vi "alu.vi"(2 "CONTROL":T3, 3 "INPUT_B":T2, 4 "INPUT_A":T2) -> (0 "OVERFLOW":bool, 1 "OUTPUT":T1)   [LabVIEW 2013]
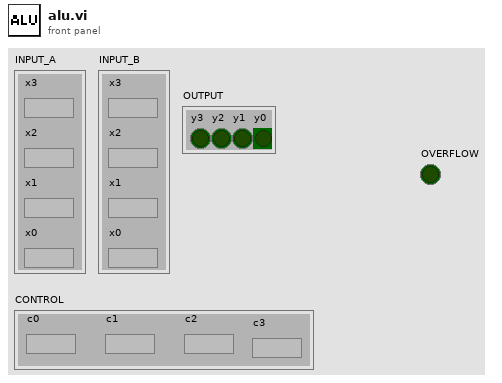
[diagram p1: front panel]
types:
  T1 = cluster{"y3":bool, "y2":bool, "y1":bool, "y0":bool}
  T2 = cluster{"x3":bool, "x2":bool, "x1":bool, "x0":bool}
  T3 = cluster{"с0":bool, "с1":bool, "с2":bool, "c3":bool}
  T4 = cluster{"y0":bool, "y1":bool, "y2":bool, "y3":bool}
  T5 = cluster{"INPUT_A":cluster{"x3":bool, "x2":bool, "x1":bool, "x0":bool}, cluster{"x3":bool, "x2":bool, "x1":bool, "x0":bool}, cluster{"x3":bool, "x2":bool, "x1":bool, "x0":bool}, cluster{"x3":bool, "x2":bool, "x1":bool, "x0":bool}, cluster{"x3":bool, "x2":bool, "x1":bool, "x0":bool}, "OUTPUT":cluster{"y3":bool, "y2":bool, "y1":bool, "y0":bool}, "OUTPUT":cluster{"y3":bool, "y2":bool, "y1":bool, "y0":bool}, "OUTPUT":cluster{"y0":bool, "y1":bool, "y2":bool, "y3":bool}, "OUTPUT":cluster{"y3":bool, "y2":bool, "y1":bool, "y0":bool}}
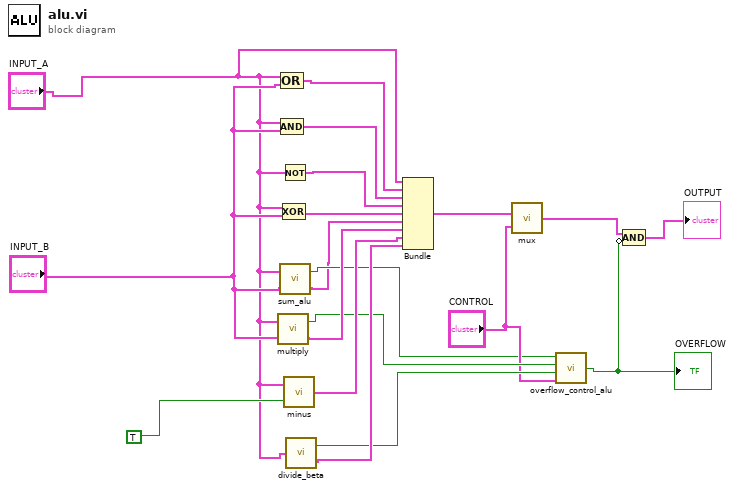
[diagram p0: block diagram]
diagram:
  n1 = call "multiply.vi"("INPUT_B"="INPUT_B", "INPUT_A"="INPUT_A") -> ("OUTPUT"=w12:T1, "OVERFLOW"=w10:bool)
  n2 = Not(x="INPUT_A") -> (.not. x?=w15:T2)
  n3 = call "sum_alu.vi"("INPUT_B"="INPUT_B", "INPUT_A"="INPUT_A") -> ("OUTPUT"=w4:T1, "OVERFLOW"=w5:bool)
  n4 = Compound Arithmetic op=OR("INPUT_A", "INPUT_B") -> (w17:T2)
  n5 = Compound Arithmetic op=AND("INPUT_A", "INPUT_B") -> (w16:T2)
  n6 = Compound Arithmetic op=XOR("INPUT_A", "INPUT_B") -> (w14:T2)
  n7 = call "minus.vi"("MINUS"=TRUE, "INPUT"="INPUT_A") -> ("OUTPUT"=w13:T4)
  n8 = call "divide_beta.vi"("INPUT"="INPUT_A") -> ("OVERFLOW"=w9:bool, "OUTPUT"=w11:T1)
  n9 = Bundle("INPUT_A"="INPUT_A", w17, w16, w15, w14, "OUTPUT"=w4, "OUTPUT"=w12, "OUTPUT"=w13, "OUTPUT"=w11) -> (w19:T5)  [unwired: 1 in]
  n10 = call "mux.vi"("CONTROL"="CONTROL", "INPUT"=w19) -> ("OUTPUT"=w1:T1)
  n11 = call "overflow_control_alu.vi"("CONTROL"="CONTROL", "over_divide"=w9, "over_multiply"=w10, "over_sum"=w5) -> ("over_flag"=w3:bool)
  "OVERFLOW" <- w3
  n12 = Compound Arithmetic op=AND(w1, invert w3) -> (→"OUTPUT":T1)
